vi "RSLT_VALUE.vi"(0 "MAX-MIN Temp":cluster{"MIN":dbl, "MAX":dbl, "ACTUAL":dbl}, 3 "INPUT cluster":T2, 5 "MAX-MIN PRESSURE":cluster{"MIN":dbl, "MAX":dbl, "ACTUALLY":dbl}, 7 "MAX-MIN FLOW":cluster{"MIN":dbl, "MAX":dbl, "ACTUALLY":dbl}, 9 "CLUSTER":T3={"Files"=[], "Browse File"=path "", "TIMEOUT"=100, "GRAPH"=[{array[68443 elements], array[68443 elements]}, {array[68363 elements], array[68363 elements]}, {array[40500 elements], array[40500 elements]}], "CHL 1"={"chl1 MIN"=110.0, "chl1 MAX"=130.0, "chl1 thrshold"=120.0}, "CHL 2"={"chl2 MIN"=33.0, "chl2 MAX"=35.0, "chl2 thrshold"=25.0}, "CHL 3"={"chl3 MIN"=20.0, "chl3 MAX"=30.0, "chl3 thrshold"=34.0}, "Report File"=path "", "Data_to_report"={"date/time string"="", "User Name"="", "BARCODE"="", "SELECTED RECIPE"="", "Rst"="", "Error Code"="", "RESULT ARRAY"=[]}, "BMP"={"chl3 MIN"=0.0, "chl3 MAX"=0.0, "chl3 thrshold"=0.0}}, 11 "error in":errorcluster, 12 "ACTUAL BPM":dbl=32134659.0 format="%#_13g") -> (4 "CLUSTER TO SQL":T1, 6 "RESULT ARRAY":string[](array[string]), 15 "error OUT":errorcluster)   [LabVIEW 2017]
panel:
  out "appended array":dbl[](array[numeric])
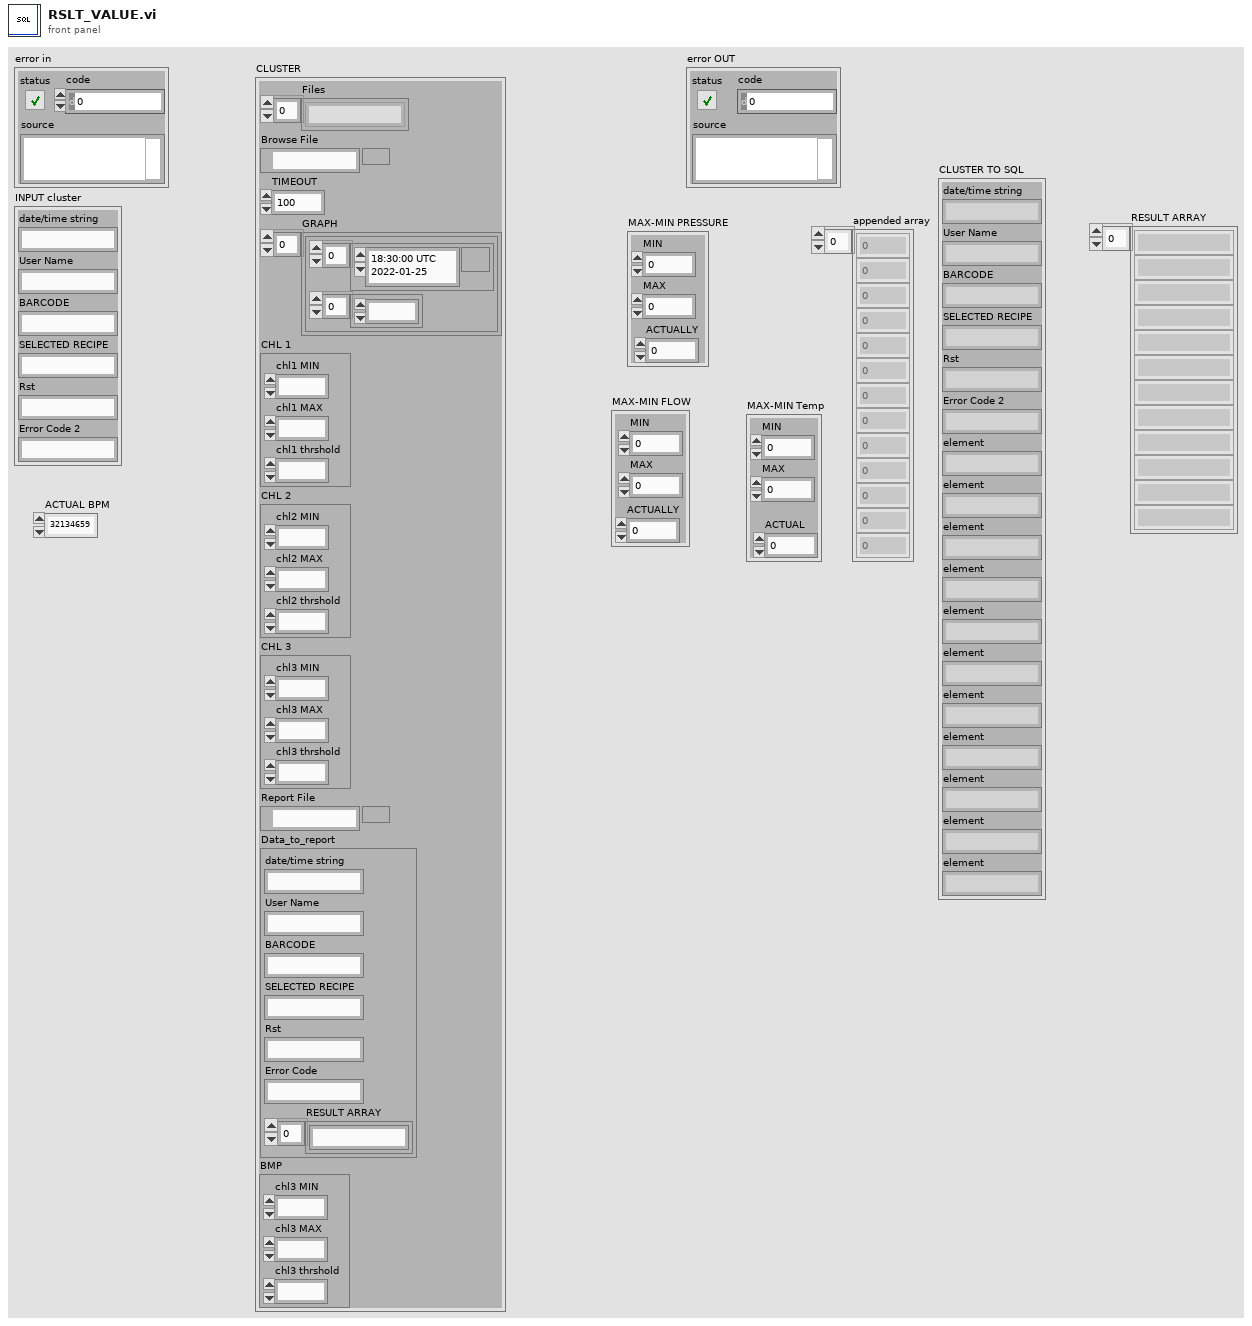
[diagram p1: front panel]
types:
  T1 = cluster{"date/time string":string, "User Name":string, "BARCODE":string, "SELECTED RECIPE":string, "Rst":string, "Error Code 2":string, "element":string, "element":string, "element":string, "element":string, "element":string, "element":string, "element":string, "element":string, "element":string, "element":string, "element":string}
  T2 = cluster{"date/time string":string, "User Name":string, "BARCODE":string, "SELECTED RECIPE":string, "Rst":string, "Error Code 2":string}
  T3 = cluster{"Files":string[], "Browse File":path, "TIMEOUT":i32, "GRAPH":cluster{timestamp[], ext[]}[], "CHL 1":cluster{"chl1 MIN":dbl, "chl1 MAX":dbl, "chl1 thrshold":dbl}, "CHL 2":cluster{"chl2 MIN":dbl, "chl2 MAX":dbl, "chl2 thrshold":dbl}, "CHL 3":cluster{"chl3 MIN":dbl, "chl3 MAX":dbl, "chl3 thrshold":dbl}, "Report File":path, "Data_to_report":cluster{"date/time string":string, "User Name":string, "BARCODE":string, "SELECTED RECIPE":string, "Rst":string, "Error Code":string, "RESULT ARRAY":string[]}, "BMP":cluster{"chl3 MIN":dbl, "chl3 MAX":dbl, "chl3 thrshold":dbl}}
  T4 = cluster{"date/time string":string, "User Name":string, "BARCODE":string, "SELECTED RECIPE":string, "Rst":string, "Error Code 2":string, "ACTUAL BPM":string, "ACTUAL BPM":string, "ACTUAL BPM":string, "ACTUAL BPM":string, "ACTUAL BPM":string, "ACTUAL BPM":string, "ACTUAL BPM":string, "ACTUAL BPM":string, "ACTUAL BPM":string, "ACTUAL BPM":string, "ACTUAL BPM":string}
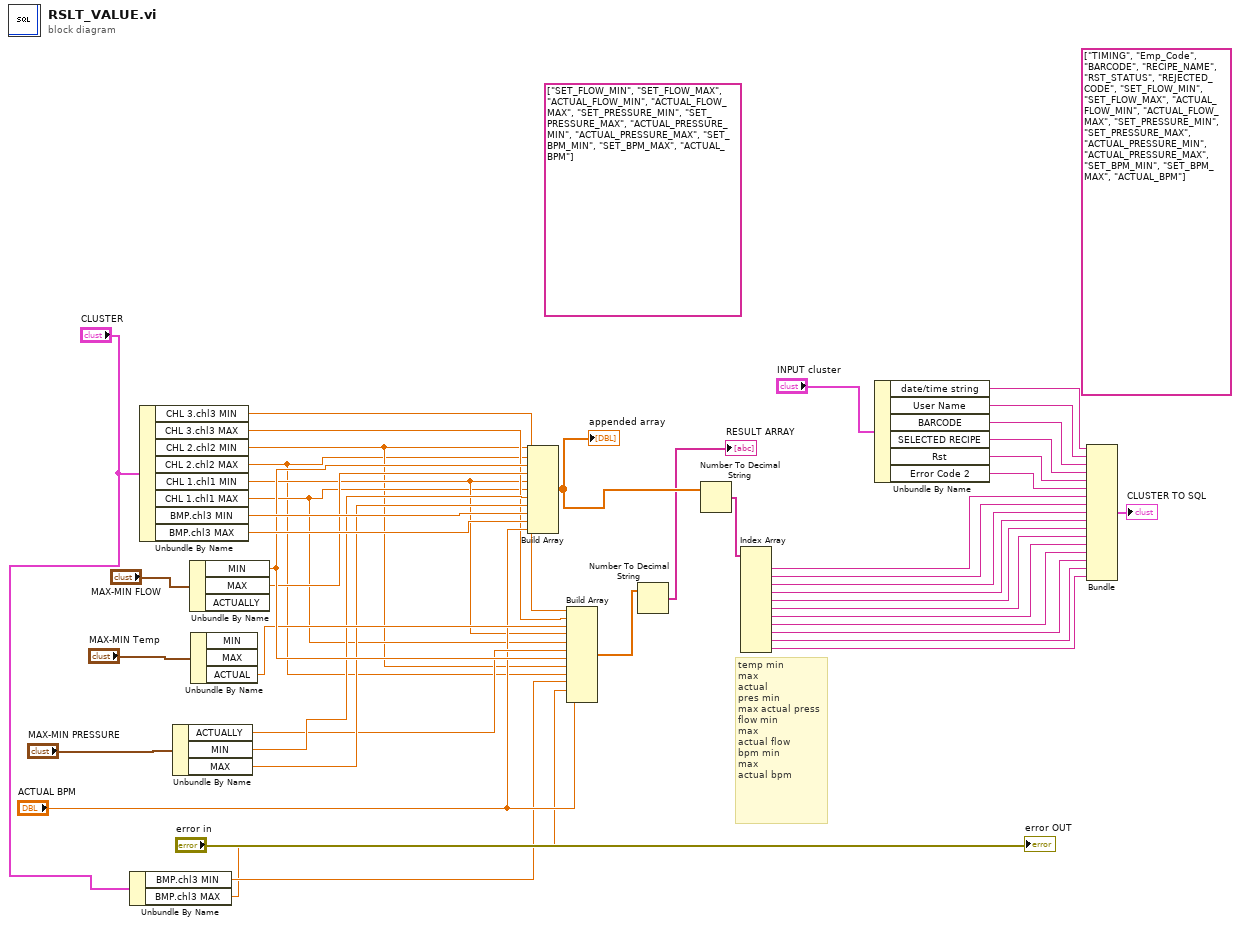
[diagram p0: block diagram]
diagram:
  (unwired) string[] ["TIMING", "Emp_Code", "BARCODE", "RECIPE_NAME", "RST_STATUS", "REJECTED_CODE", "SET_FLOW_MIN", "SET_FLOW_MAX", "ACTUAL_FLOW_MIN", "ACTUAL_FLOW_MAX", "SET_PRESSURE_MIN", "SET_PRESSURE_MAX", "ACTUAL_PRESSURE_MIN", "ACTUAL_PRESSURE_MAX", "SET_BPM_MIN", "SET_BPM_MAX", "ACTUAL_BPM"] ("columns")
  (unwired) string[] ["SET_FLOW_MIN", "SET_FLOW_MAX", "ACTUAL_FLOW_MIN", "ACTUAL_FLOW_MAX", "SET_PRESSURE_MIN", "SET_PRESSURE_MAX", "ACTUAL_PRESSURE_MIN", "ACTUAL_PRESSURE_MAX", "SET_BPM_MIN", "SET_BPM_MAX", "ACTUAL_BPM"] ("columns")
  # "temp min\nmax\nactual\npres min\nmax actual press\nflow min\nmax\nactual flow\nbpm min\nmax\nactual bpm"
  n1 = Unbundle By Name("CLUSTER") -> ("BMP.chl3 MIN"=w11:dbl, "BMP.chl3 MAX"=w10:dbl)
  n2 = Unbundle By Name("CLUSTER") -> ("CHL 3.chl3 MIN"=w6:dbl, "CHL 3.chl3 MAX"=w5:dbl, "CHL 2.chl2 MIN"=w2:dbl, "CHL 2.chl2 MAX"=w1:dbl, "CHL 1.chl1 MIN"=w4:dbl, "CHL 1.chl1 MAX"=w3:dbl, "BMP.chl3 MIN"=w42:dbl, "BMP.chl3 MAX"=w41:dbl)
  n3 = Unbundle By Name("MAX-MIN PRESSURE") -> ("ACTUALLY"=w14:dbl, "MIN"=w16:dbl, "MAX"=w15:dbl)
  n4 = Unbundle By Name("MAX-MIN FLOW") -> ("MIN"=w19:dbl, "MAX"=w18:dbl)  [unwired: 1 out]
  n5 = Unbundle By Name("MAX-MIN Temp") -> ("ACTUAL"=w17:dbl)  [unwired: 2 out]
  n6 = Build Array(w2, w1, w19, w18, w4, w3, w16, w15, w42, w41, "ACTUAL BPM") -> (w40:dbl[])
  "appended array" <- w40
  n7 = Build Array(w6, w5, w17, w4, w3, w14, w19, w2, w1, w11, w10, "ACTUAL BPM") -> (w9:dbl[])
  n8 = Number To Decimal String(number=w9) -> (decimal integer string=→"RESULT ARRAY":string[])  [unwired: 1 in]
  n9 = Number To Decimal String(number=w40) -> (decimal integer string=w8:string[])  [unwired: 1 in]
  n10 = Index Array(array=w8) -> (element #1=w31:string, element #2=w30:string, element #3=w29:string, element #4=w28:string, element #5=w27:string, element #6=w26:string, element #7=w25:string, element #8=w24:string, element #9=w23:string, element #10=w22:string, element #11=w21:string)  [unwired: 11 in]
  n11 = Unbundle By Name("INPUT cluster") -> ("date/time string"=w37:string, "User Name"=w36:string, "BARCODE"=w35:string, "SELECTED RECIPE"=w34:string, "Rst"=w33:string, "Error Code 2"=w32:string)
  n12 = Bundle("date/time string"=w37, "User Name"=w36, "BARCODE"=w35, "SELECTED RECIPE"=w34, "Rst"=w33, "Error Code 2"=w32, "ACTUAL BPM"=w31, "ACTUAL BPM"=w30, "ACTUAL BPM"=w29, "ACTUAL BPM"=w28, "ACTUAL BPM"=w27, "ACTUAL BPM"=w26, "ACTUAL BPM"=w25, "ACTUAL BPM"=w24, "ACTUAL BPM"=w23, "ACTUAL BPM"=w22, "ACTUAL BPM"=w21) -> (→"CLUSTER TO SQL":T4)  [unwired: 1 in]
  "error OUT" <- "error in"
